vi "Initialize.vi"(8 "error in (no error)":errorcluster, 11 "State in":T1={"State"=enum."Idle", "Start Time"=timestamp(0 s since 1904-01-01), "Configuration"={"Cycle Period"=0.0, "Manual Entry"=0.0, "Output Device"=enum."Default", "EPOS4 Settings"={"VISA resource name"="", "axis"={"keyHandle"=1, "nodeId"=1}, "Simulated?"=FALSE}}, "Current Time"=timestamp(0 s since 1904-01-01), "First Iteration"=FALSE, "Data"={"Centrifuge Speed"=0.0}, "Process Name"="", "Centrifuge On?"=enum."Off", "Output Error"=FALSE, "Log Started"=FALSE}) -> (0 "error out":errorcluster, 1 "Initialized":bool, 3 "State out":T1={"State"=enum."Idle", "Start Time"=timestamp(0 s since 1904-01-01), "Configuration"={"Cycle Period"=0.0, "Manual Entry"=0.0, "Output Device"=enum."Default", "EPOS4 Settings"={"VISA resource name"="", "axis"={"keyHandle"=1, "nodeId"=1}, "Simulated?"=FALSE}}, "Current Time"=timestamp(0 s since 1904-01-01), "First Iteration"=FALSE, "Data"={"Centrifuge Speed"=0.0}, "Process Name"="", "Centrifuge On?"=enum."Off", "Output Error"=FALSE, "Log Started"=FALSE})   [LabVIEW 2018, in "Centrifuge Module.lvlib" / "Centrifuge Module Engine.lvlib"]
uses:
  Centrifuge Module Engine.lvlib
  State Cluster.ctl
  State Enum.ctl
  Centrifuge Module Settings Cluster.ctl
  EPOS4/Controls/Device Selection.ctl
  EPOS4/Controls/EPOS Communication Settings.ctl
  Tag VIs/Tag FGV Operation Enum.ctl
  Shared Variables/Dynamic Shared Variables.lvlib
  EPOS4/EPOS4.lvlib
  Centrifuge Module.lvlib
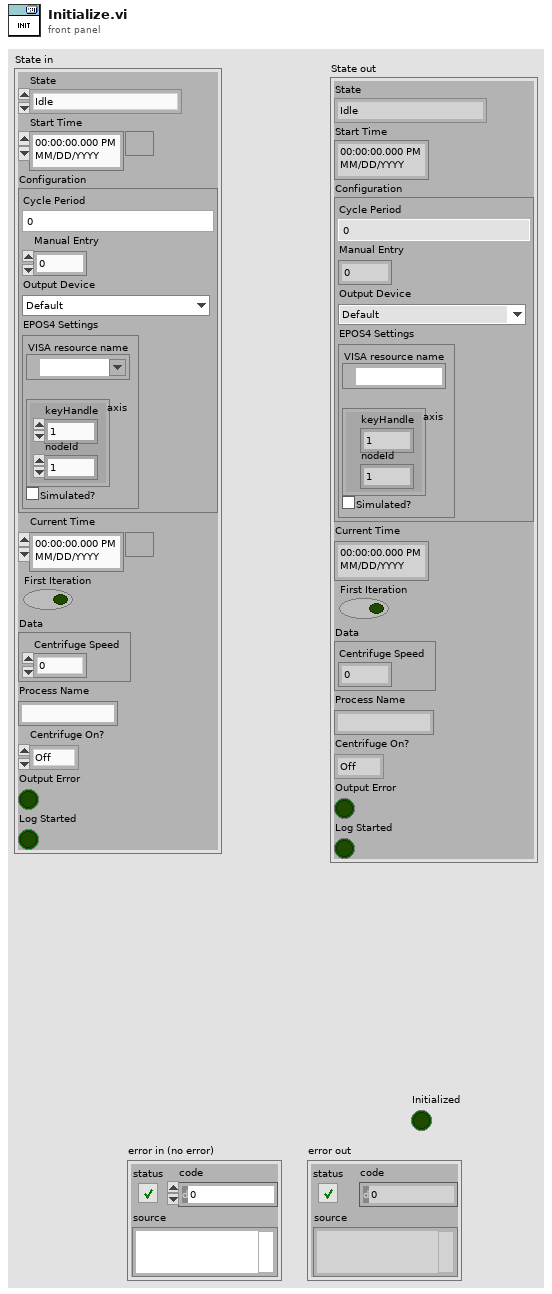
[diagram p1: front panel]
types:
  T1 = typedef "Centrifuge Module.lvlib/Centrifuge Module Engine.lvlib/State Cluster.ctl" = cluster{"State":T2, "Start Time":timestamp, "Configuration":T3, "Current Time":timestamp, "First Iteration":bool, "Data":cluster{"Centrifuge Speed":dbl}, "Process Name":string, "Centrifuge On?":enum16{"Off", "On", "Not Initialized"}, "Output Error":bool, "Log Started":bool}
  T2 = typedef "Centrifuge Module.lvlib/Centrifuge Module Engine.lvlib/State Enum.ctl" = enum16{"Measuring", "Idle", "Paused"}
  T3 = typedef "Centrifuge Module.lvlib/Centrifuge Module Settings Cluster.ctl" = cluster{"Cycle Period":dbl, "Manual Entry":dbl, "Output Device":T4, "EPOS4 Settings":T5}
  T4 = typedef "Device Selection.ctl" = enum16{"Default", "EPOS4"}
  T5 = typedef "EPOS4.lvlib/EPOS Communication Settings.ctl" = cluster{"VISA resource name":refnum<visa-resource-name>, "axis":cluster{"keyHandle":u32, "nodeId":u16}, "Simulated?":bool}
  T6 = typedef "Tag FGV Operation Enum.ctl" = enum16{"Init", "Set Notification Queue", "Create Tag", "Commit", "Write Tag (Numeric)", "Write Tag (Boolean)", "Read All Tags", "Read One Tag", "Delete Tag Category", "Set Alarm Parameters (Numeric)", "Set Alarm Parameters (Boolean)", "Enable All Alarms", "Disable All Alarms", "Delete All Tags", "Read Alarms", "Ack Alarm", "Read Alarm Parameters (Numeric)", "Read Alarm Parameters (Boolean)"}
  T7 = typedef "Centrifuge Module.lvlib/Centrifuge Module Tag Names Cluster.ctl" = cluster{"Centrifuge Speed":string, "Output Device Tag":string}
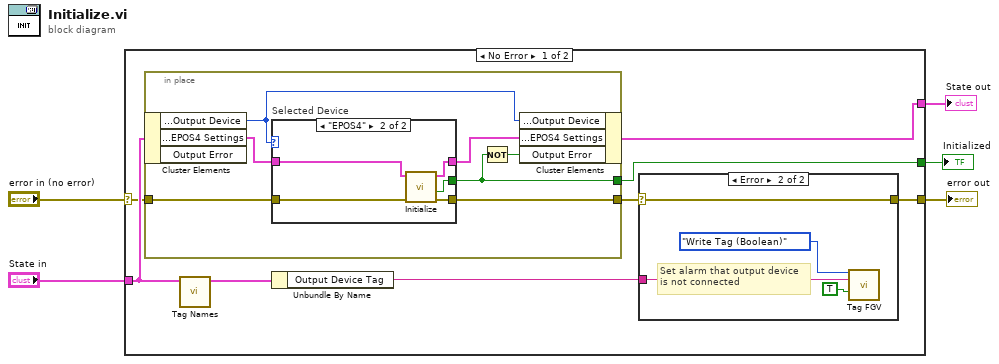
[diagram p0: block diagram]
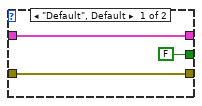
[diagram p2: hidden frame]
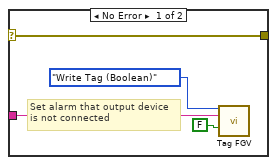
[diagram p3: hidden frame]
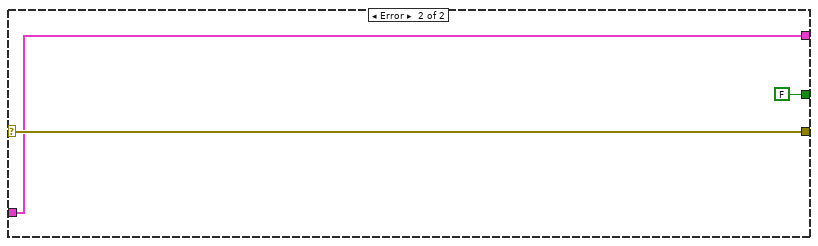
[diagram p4: hidden frame]
diagram:
  n1 = case shown="No Error" "error in (no error)" {
    selector: "error in (no error)" -> [w7 w39]
    tunnel: [w6 w39] -> w4
    tunnel: "State in" -> [w9 w38]
    tunnel: [w8 w38] -> w1
    tunnel: [w10 FALSE ("Initialized")] -> w2
    frame No Error {
      n2 = in-place {
        in-place-border: [w19] -> w13
        in-place-border: [w18] -> w10
        in-place-border: w7 -> [w15]
        n3 = in-place-cluster #1(w9) -> ("Configuration.Output Device"=w14:T4, "Configuration.EPOS4 Settings"=w17:T5)  [unwired: 1 out]
        n4 = case "Selected Device" shown="\"EPOS4\"" w14 {
          tunnel: w17 -> [w23 w28]
          tunnel: [w23 w27] -> w16
          tunnel: [w21 w25] -> w19
          tunnel: [FALSE ("Initialized") w26] -> w18
          tunnel: w15 -> [w21 w24]
          frame "Default", Default {
          }
          frame "EPOS4" {
            n5 = call "Initialize.vi"("error in (no error)"=w24, "EPOS4 Settings In"=w28) -> ("error out"=w25:errorcluster, "Initialized"=w26:bool, "EPOS4 Settings Out"=w27:T5)  [unwired: 6 in, 1 out]
          }
        }
        n6 = Not(x=w18) -> (.not. x?=w20:bool)
        n7 = in-place-cluster #1("Configuration.Output Device"=w14, "Configuration.EPOS4 Settings"=w16, "Output Error"=w20) -> (w8:T1)
      }
      n8 = call "Tag Names.vi"("State In"=w9) -> ("Centrifuge Module Tag Names"=w11:T7)  [unwired: 8 in, 2 out]
      n9 = Unbundle By Name(w11) -> ("Output Device Tag"=w12:string)
      n10 = case shown="Error" w13 {
        selector: w13 -> [w32 w36]
        tunnel: [w32 w36] -> w6
        tunnel: w12 -> [w29 w35]
        frame No Error {
          # "Set alarm that output device\nis not connected"
          n11 = call "Tag FGV.vi"("Operation"=Tag_FGV_Operation_Enum."Write Tag (Boolean)", "Tag Name"=w29, "Data"=FALSE) -> ()  [unwired: 5 in, 8 out]
        }
        frame Error {
          # "Set alarm that output device\nis not connected"
          n12 = call "Tag FGV.vi"("Operation"=Tag_FGV_Operation_Enum."Write Tag (Boolean)", "Tag Name"=w35, "Data"=TRUE) -> ()  [unwired: 5 in, 8 out]
        }
      }
    }
    frame Error {
    }
  }
  "error out" <- w4
  "State out" <- w1
  "Initialized" <- w2
